vi "MSScript_SubVI_Str&IndexToSEL.vi"(1 "Name string":cluster{"Str":string, "Start":i32}) -> (0 "SEL":cluster{"Start":u32, "End":u32}[](array[cluster]))   [LabVIEW 2018, in "MSScript.lvclass"]
uses:
  MSScript.lvclass
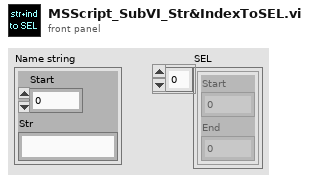
[diagram p1: front panel]
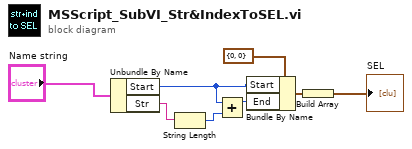
[diagram p0: block diagram]
diagram:
  n1 = Unbundle By Name("Name string") -> ("Start"=w6:i32, "Str"=w2:string)
  n2 = String Length(string=w2) -> (length=w3:i32)
  n3 = Add(x=w6, y=w3) -> (x+y=w4:i32)
  n4 = Bundle By Name(cluster=cluster{"Start":u32, "End":u32} {"Start"=0, "End"=0}, "Start"=w6, "End"=w4) -> (w7:cluster{"Start":u32, "End":u32})
  n5 = Build Array(w7) -> (→"SEL":cluster{"Start":u32, "End":u32}[])
